vi "Get Template Message Path.vi"(8 "error in":errorcluster, 10 "Message Type":T1, 11 "Message Recipient Type":T2) -> (0 "error out":errorcluster, 2 "appended path":path)   [LabVIEW 2023, in "Message Maker.lvclass"]
doc: "Fets the path of the message template class"
uses:
  Message Maker.lvclass
  Message Recipient Type.ctl
  Message Type.ctl
  <vilib>/Utility/error.llb/Error Cluster From Error Code.vi
  <vilib>/ErrorRing/Error Ring.xnode
  Message Maker.lvclass/Message Maker.ctl
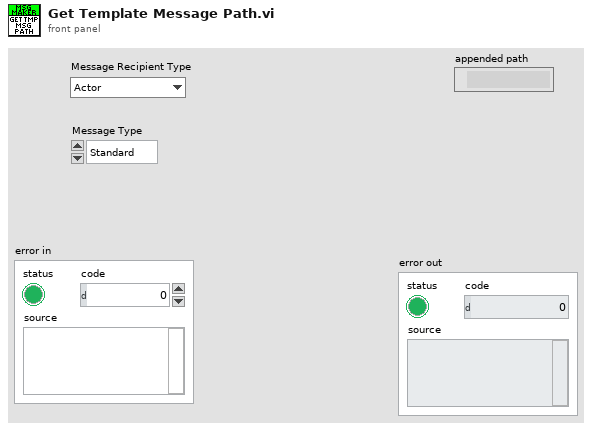
[diagram p1: front panel]
types:
  T1 = typedef "Message Maker.lvclass/Message Type.ctl" = enum16{"Standard", "Async"}
  T2 = typedef "Message Maker.lvclass/Message Recipient Type.ctl" = enum16{"Actor", "Interface", "Async Actor"}
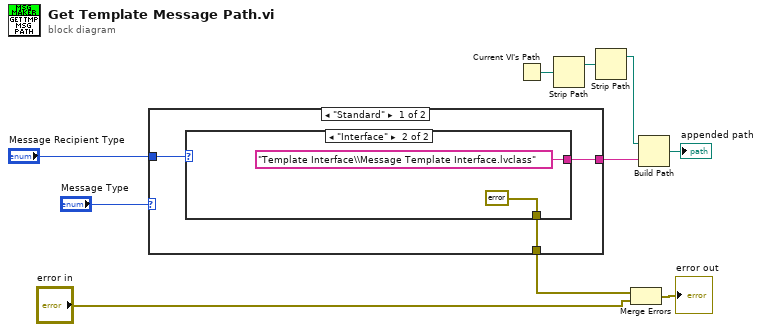
[diagram p0: block diagram]
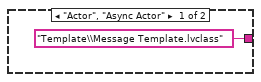
[diagram p2: hidden frame]
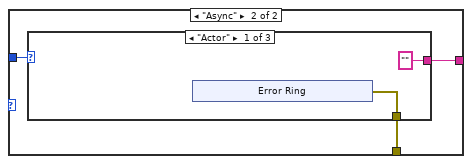
[diagram p3: hidden frame]
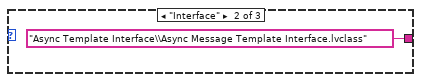
[diagram p4: hidden frame]
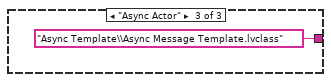
[diagram p5: hidden frame]
diagram:
  n1 = case shown="\"Standard\"" "Message Type" {
    tunnel: [w13 w19] -> w9
    tunnel: "Message Recipient Type" -> [w12 w18]
    tunnel: [w11 w17] -> w3
    frame "Standard" {
      n2 = case shown="\"Interface\"" w12 {
        tunnel: ["Template\\Message Template.lvclass" ("name or relative path") "Template Interface\\Message Template Interface.lvclass" ("name or relative path")] -> w13
        tunnel: [_ errorcluster {"status"=FALSE, "code"=0, "source"=""} ("error out")] -> w11
        frame "Actor", "Async Actor" {
        }
        frame "Interface" {
        }
      }
    }
    frame "Async" {
      n3 = case shown="\"Actor\"" w18 {
        tunnel: ["" ("name or relative path") "Async Template Interface\\Async Message Template Interface.lvclass" ("name or relative path") "Async Template\\Async Message Template.lvclass" ("name or relative path")] -> w19
        tunnel: [w20 _ _] -> w17
        frame "Actor" {
          n4 = xnode "Error Ring"() -> ("error out"=w20:errorcluster)
        }
        frame "Interface" {
        }
        frame "Async Actor" {
        }
      }
    }
  }
  n5 = Current VI's Path() -> (path=w8:path)
  n6 = Strip Path(path=w8) -> (stripped path=w7:path)  [unwired: 1 out]
  n7 = Strip Path(path=w7) -> (stripped path=w6:path)  [unwired: 1 out]
  n8 = Merge Errors(w3, "error in") -> (→"error out":errorcluster)
  n9 = Build Path(base path=w6, name or relative path=w9) -> (appended path=→"appended path":path)
